vi "Comm_Write.vi"(8 "error in (no error)":errorcluster, 9 "Text to write":string, 11 "Python":T1) -> (0 "error out":errorcluster, 2 "reply":string)   [LabVIEW 2022 SP3]
uses:
  PythonCtrl.ctl
  Processors.ctl
panel:
  out "result string":string
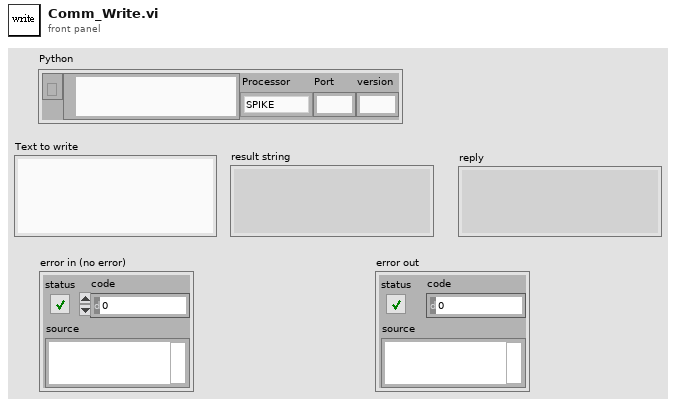
[diagram p1: front panel]
types:
  T1 = typedef "PythonCtrl.ctl" = cluster{"session":refnum<k35>, "PyPath":path, "Processor":T2, "Port":string, "version":string}
  T2 = typedef "Processors.ctl" = enum16{"SPIKE", "Pi", "Pi_ssh", "OpenMV", "Dunio"}
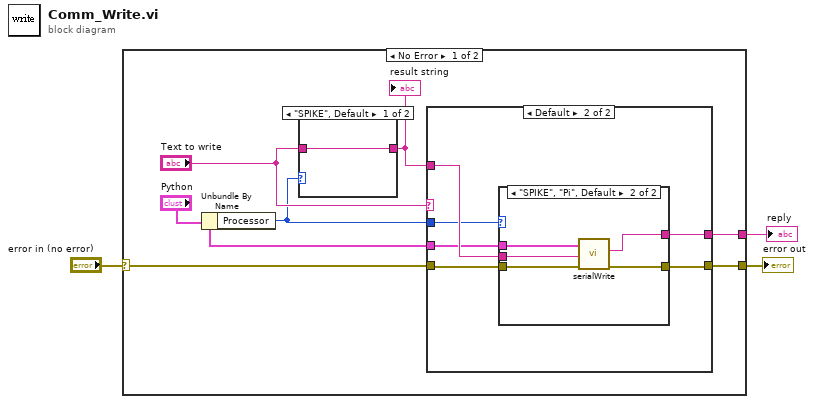
[diagram p0: block diagram]
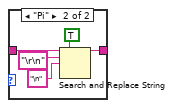
[diagram p2: hidden frame]
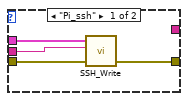
[diagram p4: hidden frame]
diagram:
  n1 = case shown="No Error" "error in (no error)" {
    selector: "error in (no error)" -> [w5 w33]
    tunnel: [w10 w33] -> w3
    tunnel: [w4 _] -> w1
    frame No Error {
      n2 = Unbundle By Name("Python") -> ("Processor"=w6:T2)
      n3 = case shown="\"SPIKE\", Default" w6 {
        tunnel: "Text to write" -> [w11 w16]
        tunnel: [w11 w15] -> w8
        frame "SPIKE", Default {
        }
        frame "Pi" {
          n4 = Search and Replace String(replace all?=TRUE ("replace all? (F)"), input string=w16, search string="\r\n" ("regular expression"), replace string="\n" ("regular expression")) -> (result string=w15:string)  [unwired: 4 in, 3 out]
        }
      }
      "result string" <- w8
      n5 = case shown="Default" "Text to write" {
        tunnel: w8 -> [_ w23]
        tunnel: w5 -> [w17 w22]
        tunnel: [w17 w21] -> w10
        tunnel: "Python" -> [_ w20]
        tunnel: w6 -> [_ w19]
        tunnel: [_ w18] -> w4
        frame "" {
        }
        frame Default {
          n6 = case shown="\"SPIKE\", \"Pi\", Default" w19 {
            tunnel: w23 -> [w24 w29]
            tunnel: w22 -> [w27 w32]
            tunnel: [w26 w31] -> w21
            tunnel: w20 -> [w25 w30]
            tunnel: [_ w28] -> w18
            frame "Pi_ssh" {
              n7 = call "SSH_Write.vi"("error in (no error)"=w27, "Text to write"=w24, "Python"=w25) -> ("error out"=w26:errorcluster)  [unwired: 7 in, 1 out]
            }
            frame "SPIKE", "Pi", Default {
              n8 = call "serialWrite.vi"("error in (no error)"=w32, "text"=w29, "Python"=w30) -> ("error out"=w31:errorcluster, "reply"=w28:string)  [unwired: 6 in, 1 out]
            }
          }
        }
      }
    }
    frame Error {
    }
  }
  "error out" <- w3
  "reply" <- w1
